vi "ESC_StdSci_WorkBench.vi"() -> ()   [LabVIEW 2015]
uses:
  SCI_DataPck.ctl
  SCI_DataType.ctl
panel:
  out "串口读缓存字符数":u32
  in  "VISA资源名称":refnum<visa-resource-name>="COM1"
  out "串口读数据":i32[](array[numeric]) format="%04x"
  out "串口缓存非空":bool
  out "串口写入数据":string
  out "串口读数据包":T1={"包头"=170, "数据低8位"=0, "数据低高8位"=0, "数据类型"=0, "CRC余数"=0, "数据无效"=FALSE, "数据更新"=FALSE} {"包头" format="%02x"; "数据低8位" format="%02x"; "数据低高8位" format="%02x"; "数据类型" items=["SCIDP_SPTG1"=16, "SCIDP_SPTG2"=17, "SCIDP_INSTR1"=18, "SCIDP_INSTR2"=19, "SCIDP_DTTG1"=20, "SCIDP_DTTG2"=21, "SCIDP_VRPH1"=22, "SCIDP_VRPH2"=23, "RSVD0x18"=24, "RSVD0x19"=25, "RSVD0x1A"=26, "RSVD0x1B"=27, "RSVD0x1C"=28, "RSVD0x1D"=29, "RSVD0x1E"=30, "RSVD0x1F"=31, "SCIDP_SRVST1"=32, "SCIDP_SRVST2"=33, "SCIDP_SPFB1"=34, "SCIDP_SPFB2"=35, "RSVD0x24"=36, "RSVD0x25"=37, "RSVD0x26"=38, "RSVD0x27"=39, "RSVD0x28"=40, "RSVD0x29"=41, "RSVD0x2A"=42, "RSVD0x2B"=43, "RSVD0x2C"=44, "RSVD0x2D"=45, "SCIDP_EFFC1"=46, "SCIDP_EFFC2"=47, "RSVD0x30"=48, "RSVD0x31"=49, "SCIDP_IBUS1"=50, "SCIDP_IBUS2"=51, "SCIDP_IA1"=52, "SCIDP_IA2"=53, "SCIDP_IB1"=54, "SCIDP_IB2"=55, "SCIDP_IC1"=56, "SCIDP_IC2"=57, "SCIDP_UBUS1"=58, "SCIDP_UBUS2"=59, "SCIDP_TMPR1"=60, "SCIDP_TMPR2"=61, "RSVD0x3E"=62, "RSVD0x3F"=63, "VOID"=0]; "CRC余数" format="%02x"}
  out "串口预写入簇":T1={"包头"=170, "数据低8位"=0, "数据低高8位"=0, "数据类型"=0, "CRC余数"=0, "数据无效"=FALSE, "数据更新"=FALSE} {"包头" format="%02x"; "数据低8位" format="%02x"; "数据低高8位" format="%02x"; "数据类型" items=["SCIDP_SPTG1"=16, "SCIDP_SPTG2"=17, "SCIDP_INSTR1"=18, "SCIDP_INSTR2"=19, "SCIDP_DTTG1"=20, "SCIDP_DTTG2"=21, "SCIDP_VRPH1"=22, "SCIDP_VRPH2"=23, "RSVD0x18"=24, "RSVD0x19"=25, "RSVD0x1A"=26, "RSVD0x1B"=27, "RSVD0x1C"=28, "RSVD0x1D"=29, "RSVD0x1E"=30, "RSVD0x1F"=31, "SCIDP_SRVST1"=32, "SCIDP_SRVST2"=33, "SCIDP_SPFB1"=34, "SCIDP_SPFB2"=35, "RSVD0x24"=36, "RSVD0x25"=37, "RSVD0x26"=38, "RSVD0x27"=39, "RSVD0x28"=40, "RSVD0x29"=41, "RSVD0x2A"=42, "RSVD0x2B"=43, "RSVD0x2C"=44, "RSVD0x2D"=45, "SCIDP_EFFC1"=46, "SCIDP_EFFC2"=47, "RSVD0x30"=48, "RSVD0x31"=49, "SCIDP_IBUS1"=50, "SCIDP_IBUS2"=51, "SCIDP_IA1"=52, "SCIDP_IA2"=53, "SCIDP_IB1"=54, "SCIDP_IB2"=55, "SCIDP_IC1"=56, "SCIDP_IC2"=57, "SCIDP_UBUS1"=58, "SCIDP_UBUS2"=59, "SCIDP_TMPR1"=60, "SCIDP_TMPR2"=61, "RSVD0x3E"=62, "RSVD0x3F"=63, "VOID"=0]; "CRC余数" format="%02x"}
  out "写数据更新":bool
  in  "串口写数据包":T1={"包头"=170, "数据低8位"=0, "数据低高8位"=0, "数据类型"=0, "CRC余数"=0, "数据无效"=FALSE, "数据更新"=FALSE} {"包头" format="%02x"; "数据低8位" format="%02x"; "数据低高8位" format="%02x"; "数据类型" items=["SCIDP_SPTG1"=16, "SCIDP_SPTG2"=17, "SCIDP_INSTR1"=18, "SCIDP_INSTR2"=19, "SCIDP_DTTG1"=20, "SCIDP_DTTG2"=21, "SCIDP_VRPH1"=22, "SCIDP_VRPH2"=23, "RSVD0x18"=24, "RSVD0x19"=25, "RSVD0x1A"=26, "RSVD0x1B"=27, "RSVD0x1C"=28, "RSVD0x1D"=29, "RSVD0x1E"=30, "RSVD0x1F"=31, "SCIDP_SRVST1"=32, "SCIDP_SRVST2"=33, "SCIDP_SPFB1"=34, "SCIDP_SPFB2"=35, "RSVD0x24"=36, "RSVD0x25"=37, "RSVD0x26"=38, "RSVD0x27"=39, "RSVD0x28"=40, "RSVD0x29"=41, "RSVD0x2A"=42, "RSVD0x2B"=43, "RSVD0x2C"=44, "RSVD0x2D"=45, "SCIDP_EFFC1"=46, "SCIDP_EFFC2"=47, "RSVD0x30"=48, "RSVD0x31"=49, "SCIDP_IBUS1"=50, "SCIDP_IBUS2"=51, "SCIDP_IA1"=52, "SCIDP_IA2"=53, "SCIDP_IB1"=54, "SCIDP_IB2"=55, "SCIDP_IC1"=56, "SCIDP_IC2"=57, "SCIDP_UBUS1"=58, "SCIDP_UBUS2"=59, "SCIDP_TMPR1"=60, "SCIDP_TMPR2"=61, "RSVD0x3E"=62, "RSVD0x3F"=63, "VOID"=0]; "CRC余数" format="%02x"}
  in  "写入数据 2":u16 format="%x"
  in  "写入数据类型 2":u16 format="%x"
  in  "发送 2":bool
  out "写数据CRC余数 2":u16 format="%x"
  in  "停止按钮":bool
  out "串口更新":bool=TRUE
  out "串口缓存空":bool
  in  "读出数据类型":u16=16 format="%02x"
  out "读数据CRC余数":u16 format="%x"
  out "读出数据":u16 format="%x"
  out "包头":u16 format="%x"
  in  "写入数据 1":u16 format="%x"
  in  "写入数据类型 1":u16 format="%x"
  in  "发送 1":bool
  out "写数据CRC余数 1":u16 format="%x"
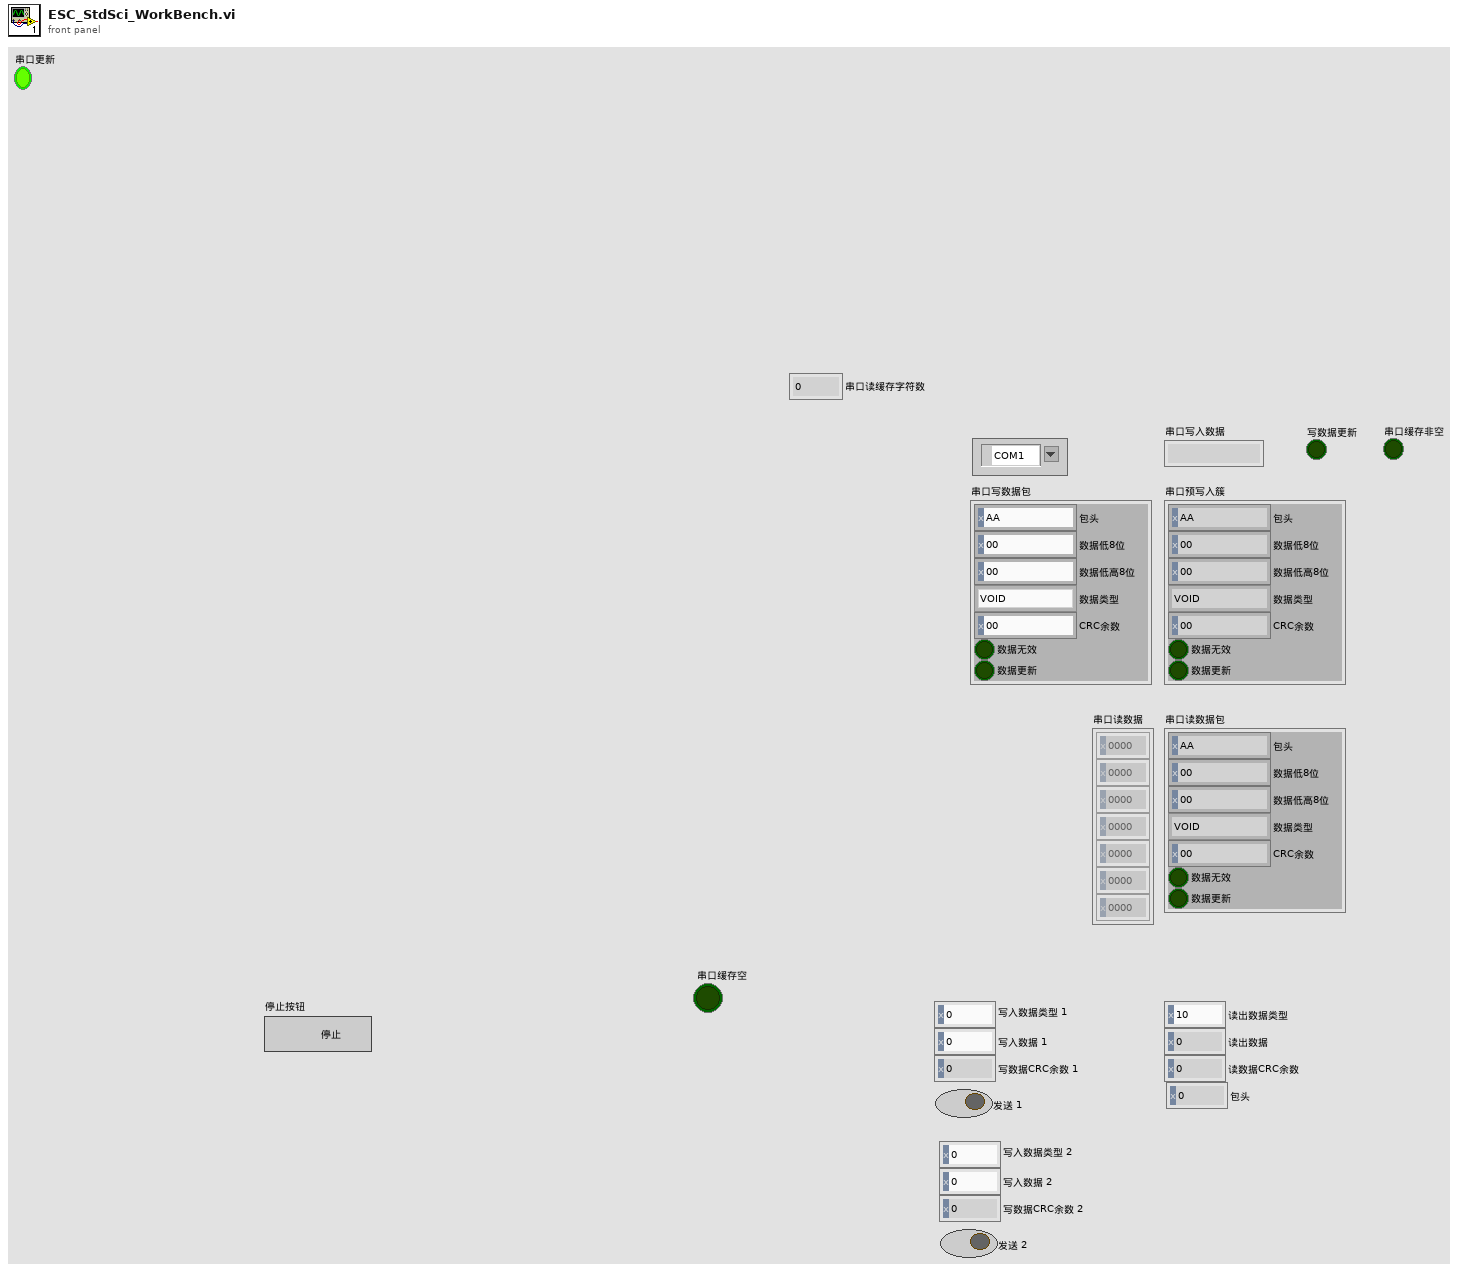
[diagram p1: front panel]
types:
  T1 = typedef "SCI_DataPck.ctl" = cluster{"包头":u16, "数据低8位":u16, "数据低高8位":u16, "数据类型":T2, "CRC余数":u16, "数据无效":bool, "数据更新":bool}
  T2 = typedef "SCI_DataType.ctl" = u16
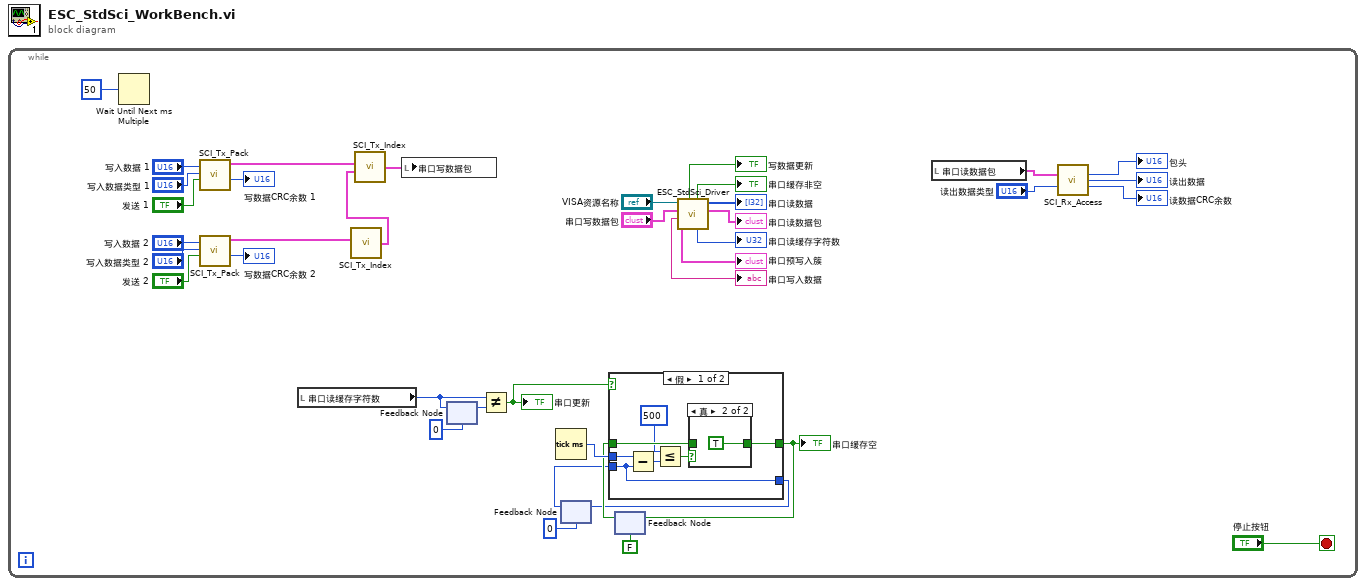
[diagram p0: block diagram]
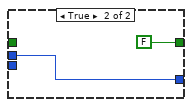
[diagram p3: hidden frame]
diagram:
  n1 = while {
    stop <- "停止按钮" stop-if-true
    n2 = Wait Until Next ms Multiple(millisecond multiple=50) -> ()  [unwired: 1 out]
    n3 = call "SCI_Tx_Pack.vi"("数据有效"="发送 1", "数据类型"="写入数据类型 1", "数据"="写入数据 1") -> ("CRC余数"=→"写数据CRC余数 1":u16, "数据包输出"=w5:T1)  [unwired: 7 in]
    n4 = call "SCI_Tx_Pack.vi"("数据有效"="发送 2", "数据类型"="写入数据类型 2", "数据"="写入数据 2") -> ("CRC余数"=→"写数据CRC余数 2":u16, "数据包输出"=w6:T1)  [unwired: 7 in]
    n5 = local read "串口读缓存字符数"() -> (w21:u32)
    n6 = call "SCI_Tx_Index.vi"("输入数据包（簇）"=w6) -> ("上一个包数据（簇）"=w3:T1)  [unwired: 6 in]
    n7 = call "SCI_Tx_Index.vi"("输入数据包（簇）"=w5, "下一包数据（簇）"=w3) -> ("上一个包数据（簇）"=w4:T1)  [unwired: 5 in]
    n8 = local write "串口写数据包"(w4) -> ()
    n9 = feedback #1(u32 0 ("Bytes at Port")) -> (w29:u32)
    n10 = feedback-in #1(w21) -> ()
    n11 = Not Equal?(x=w21, y=w29) -> (x != y?=w36:bool)
    "串口更新" <- w36
    n12 = Tick Count (ms)() -> (millisecond timer value=w37:u32)
    n13 = feedback #2(u32 0 ("Bytes at Port")) -> (w22:u32)
    n14 = feedback #3(FALSE) -> (w25:bool)
    n15 = case shown="假" w36 {
      tunnel: [w44 w50] -> w23
      tunnel: w37 -> [w46 w50]
      tunnel: w22 -> [w44 _]
      tunnel: [w42 FALSE ("crossing")] -> w26
      tunnel: w25 -> [w43 _]
      frame False {
        n16 = Subtract(x=w46, y=w44) -> (x-y=w41:u32)
        n17 = Less Or Equal?(x=500, y=w41) -> (x <= y?=w45:bool)
        n18 = case shown="真" w45 {
          tunnel: w43 -> [w47 _]
          tunnel: [w47 TRUE ("crossing")] -> w42
          frame False {
          }
          frame True {
          }
        }
      }
      frame True {
      }
    }
    "串口缓存空" <- w26
    n19 = feedback-in #2(w23) -> ()
    n20 = feedback-in #3(w26) -> ()
    n21 = call "ESC_StdSci_Driver.vi"("串口写数据包"="串口写数据包", "VISA资源名称"="VISA资源名称") -> ("串口读数据包"=→"串口读数据包":T1, "串口读数据"=→"串口读数据":i32[], "串口读缓存字符数"=→"串口读缓存字符数":u32, "串口缓存非空"=→"串口缓存非空":bool, "写数据更新"=→"写数据更新":bool, "串口写入数据包"=→"串口预写入簇":T1, "串口写入数据"=→"串口写入数据":string)  [unwired: 3 in]
    n22 = local read "串口读数据包"() -> (w16:T1)
    n23 = call "SCI_Rx_Access.vi"("串口读数据包（簇）"=w16, "数据类型"="读出数据类型") -> ("包头"=→"包头":u16, "数据输出"=→"读出数据":u16, "CRC余数"=→"读数据CRC余数":u16)  [unwired: 11 in]
  }
